vi "Insert_Into_Array_2D.vi"(9 "SubArray IIA 2D":i8[][](array[numeric]), 10 "Indexs IIA":T1, 11 "Insert Into Array 2D":i8[][](array[numeric])) -> (3 "Array 2D IIA":i8[][](array[numeric]))   [LabVIEW 2018]
uses:
  Controls/Rows_Columns.ctl
panel:
  out "IRR":i32
  out "ICC":i32
  out "SC":i32
  out "SR":i32
  out "IRC":i32
  out "SC1":i32
  out "SR1":i32
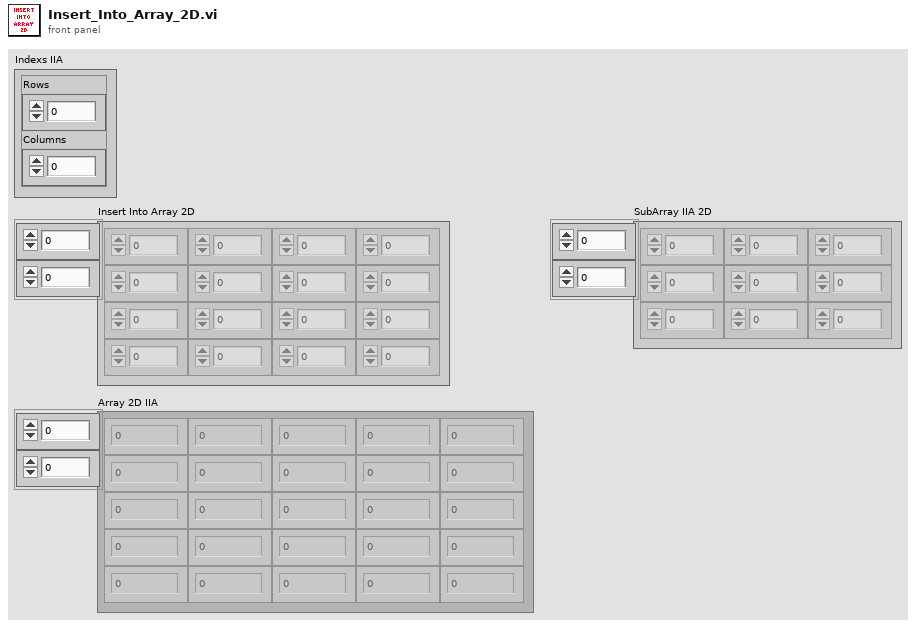
[diagram p1: front panel]
types:
  T1 = typedef "Rows_Columns.ctl" = cluster{"Rows":i32, "Columns":i32}
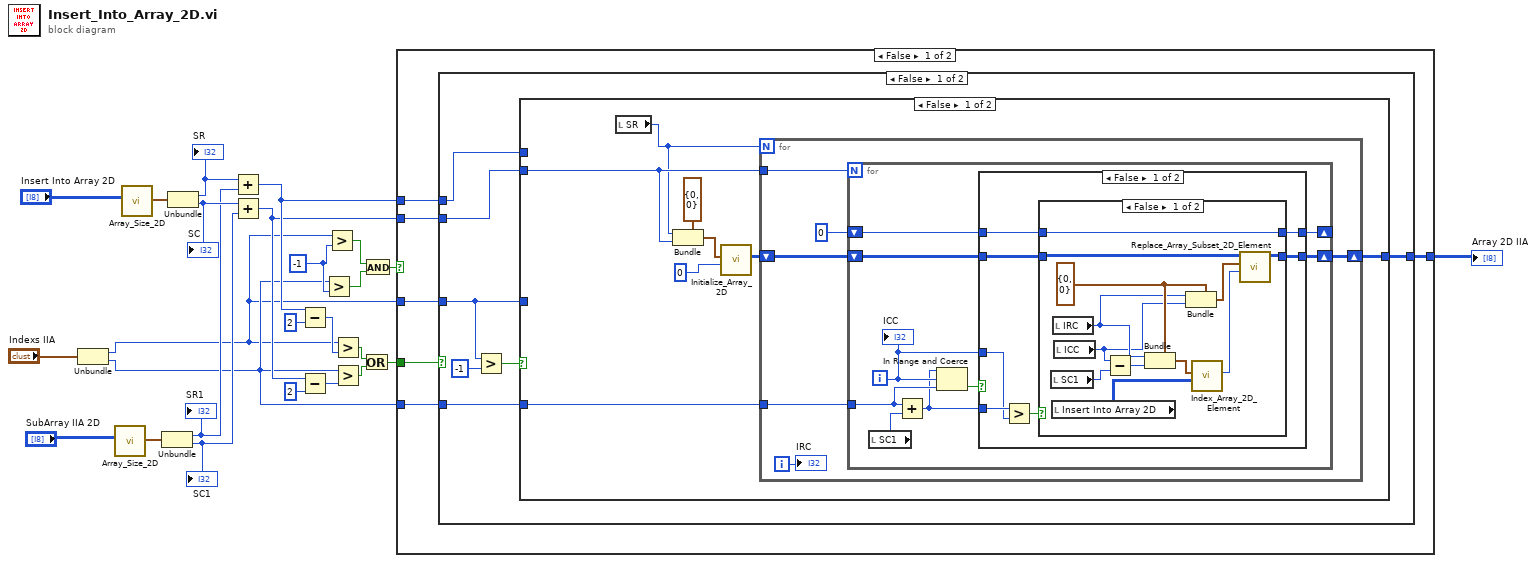
[diagram p0: block diagram]
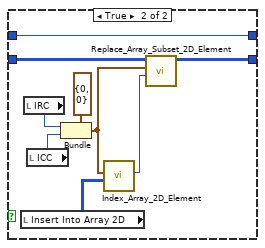
[diagram p2: hidden frame]
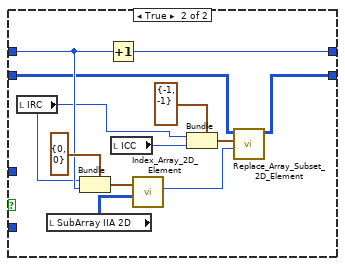
[diagram p3: hidden frame]
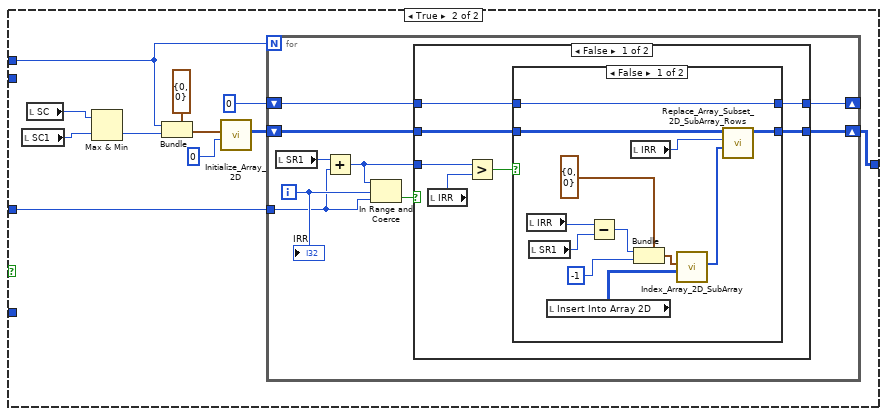
[diagram p4: hidden frame]
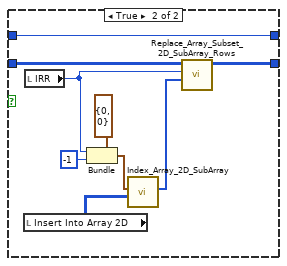
[diagram p5: hidden frame]
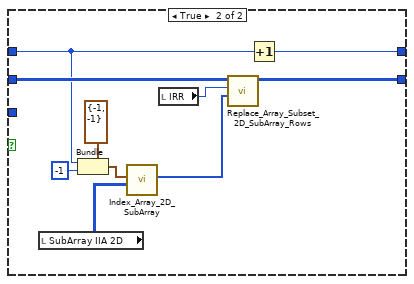
[diagram p6: hidden frame]
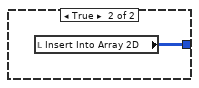
[diagram p7: hidden frame]
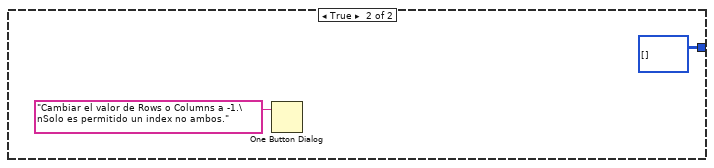
[diagram p8: hidden frame]
diagram:
  w3 = -1 ("y")
  n1 = Unbundle("Indexs IIA") -> ("Rows"=w1:i32, "Columns"=w2:i32)
  n2 = call "Array_Size_2D.vi"("Array"="SubArray IIA 2D") -> ("Size 2D"=w23:T1)  [unwired: 10 in]
  n3 = call "Array_Size_2D.vi"("Array"="Insert Into Array 2D") -> ("Size 2D"=w24:T1)  [unwired: 10 in]
  n4 = Unbundle(w23) -> ("Rows"=w10:i32, "Columns"=w21:i32)
  "SR1" <- w10
  "SC1" <- w21
  n5 = Unbundle(w24) -> ("Rows"=w11:i32, "Columns"=w22:i32)
  "SR" <- w11
  "SC" <- w22
  n6 = Add(x=w11, y=w10) -> (x+y=w18:i32)
  n7 = Add(x=w22, y=w21) -> (x+y=w9:i32)
  n8 = Subtract(x=w18, y=2) -> (x-y=w16:i32)
  n9 = Subtract(x=w9, y=2) -> (x-y=w14:i32)
  n10 = Greater?(x=w2, y=w3) -> (0:w4:bool)
  n11 = Greater?(x=w1, y=w3) -> (0:w5:bool)
  n12 = Greater?(x=w1, y=w16) -> (0:w20:bool)
  n13 = Greater?(x=w2, y=w14) -> (0:w19:bool)
  n14 = Or(x=w20, y=w19) -> (x .or. y?=w12:bool)
  n15 = And(x=w5, y=w4) -> (x .and. y?=w6:bool)
  n16 = case shown="False" w6 {
    tunnel: w18 -> [w31 _]
    tunnel: w12 -> [w30 _]
    tunnel: w9 -> [w29 _]
    tunnel: w2 -> [w28 _]
    tunnel: w1 -> [w27 _]
    tunnel: [w26 i8[][] [] ("Insert Into Array 2D")] -> w7
    frame False {
      n17 = case shown="False" w30 {
        tunnel: w31 -> [w35 _]
        tunnel: w27 -> [w33 _]
        tunnel: w28 -> [w34 _]
        tunnel: w29 -> [w36 _]
        tunnel: [w32 w160] -> w26
        frame False {
          n18 = Greater?(x=w33, y=-1) -> (0:w37:bool)
          n19 = case shown="False" w37 {
            tunnel: w36 -> [w45 _]
            tunnel: w35 -> [_ w106]
            tunnel: w34 -> [w46 _]
            tunnel: w33 -> [_ w108]
            tunnel: [w40 w105] -> w32
            frame False {
              n20 = local read "SR"() -> (w39:i32)
              n21 = Bundle(cluster=T1 {"Rows"=0, "Columns"=0} ("Dimensions"), "Rows"=w39, "Columns"=w45) -> (w42:T1)
              n22 = call "Initialize_Array_2D.vi"("Value"=i8 0, "Dimensions"=w42) -> ("Initialized Array 2D"=w41:i8[][])  [unwired: 9 in]
              n23 = for {
                N: w39 -> [_]
                tunnel: w45 -> [w51]
                shift-right: [w47] -> w40
                shift-left: w41 -> [w49]
                tunnel: w46 -> [w50]
                i -> [w52]
                n24 = for {
                  N: w51 -> [_]
                  tunnel: w50 -> [w61]
                  shift-right: [w55] -> _
                  shift-left: 0 -> [w56]
                  shift-right: [w53] -> w47
                  shift-left: w49 -> [w54]
                  i -> [w58]
                  n25 = local read "SC1"() -> (w60:i32)
                  n26 = Add(x=w61, y=w60) -> (x+y=w57:i32)
                  n27 = In Range and Coerce(upper limit=w57, x=w58, lower limit=w61) -> (In Range?=w59:bool)  [unwired: 1 out]
                  n28 = case shown="False" w59 {
                    tunnel: w58 -> [w67 _]
                    tunnel: w57 -> [w68 _]
                    tunnel: [w64 w101] -> w55
                    tunnel: w56 -> [w65 w99]
                    tunnel: w54 -> [w62 w94]
                    tunnel: [w63 w95] -> w53
                    frame False {
                      n29 = Greater?(x=w68, y=w67) -> (0:w66:bool)
                      n30 = case shown="False" w66 {
                        tunnel: [w80 w89] -> w64
                        tunnel: w65 -> [w80 w89]
                        tunnel: [w79 w88] -> w63
                        tunnel: w62 -> [w78 w87]
                        frame False {
                          w74 = T1 {"Rows"=0, "Columns"=0} ("Indexs IA")
                          n31 = local read "SC1"() -> (w72:i32)
                          n32 = local read "Insert Into Array 2D"() -> (w77:i8[][])
                          n33 = local read "IRC"() -> (w73:i32)
                          n34 = local read "ICC"() -> (w70:i32)
                          n35 = Subtract(x=w70, y=w72) -> (x-y=w71:i32)
                          n36 = Bundle(cluster=w74, "Rows"=w73, "Columns"=w71) -> (w69:T1)
                          n37 = Bundle(cluster=w74, "Rows"=w73, "Columns"=w70) -> (w75:T1)
                          n38 = call "Index_Array_2D_Element.vi"("Index Array 2D"=w77, "Indexs IA"=w69) -> ("Value"=w76:i8)  [unwired: 9 in]
                          n39 = call "Replace_Array_Subset_2D_Element.vi"("Element RAS"=w76, "Indexs RAS"=w75, "RAS2D"=w78) -> ("New Array RAS2D"=w79:i8[][])  [unwired: 8 in]
                        }
                        frame True {
                          n40 = local read "Insert Into Array 2D"() -> (w85:i8[][])
                          n41 = local read "IRC"() -> (w82:i32)
                          n42 = local read "ICC"() -> (w83:i32)
                          n43 = Bundle(cluster=T1 {"Rows"=0, "Columns"=0} ("Indexs IA"), "Rows"=w82, "Columns"=w83) -> (w81:T1)
                          n44 = call "Index_Array_2D_Element.vi"("Index Array 2D"=w85, "Indexs IA"=w81) -> ("Value"=w86:i8)  [unwired: 9 in]
                          n45 = call "Replace_Array_Subset_2D_Element.vi"("Element RAS"=w86, "Indexs RAS"=w81, "RAS2D"=w87) -> ("New Array RAS2D"=w88:i8[][])  [unwired: 8 in]
                        }
                      }
                    }
                    frame True {
                      n46 = local read "IRC"() -> (w90:i32)
                      n47 = local read "SubArray IIA 2D"() -> (w97:i8[][])
                      n48 = Bundle(cluster=T1 {"Rows"=0, "Columns"=0} ("Indexs IA"), "Rows"=w90, "Columns"=w99) -> (w98:T1)
                      n49 = Increment(x=w99) -> (x+1=w101:i32)
                      n50 = local read "ICC"() -> (w91:i32)
                      n51 = call "Index_Array_2D_Element.vi"("Index Array 2D"=w97, "Indexs IA"=w98) -> ("Value"=w96:i8)  [unwired: 9 in]
                      n52 = Bundle(cluster=T1 {"Rows"=-1, "Columns"=-1} ("Rows & Columns"), "Rows"=w90, "Columns"=w91) -> (w92:T1)
                      n53 = call "Replace_Array_Subset_2D_Element.vi"("Element RAS"=w96, "Indexs RAS"=w92, "RAS2D"=w94) -> ("New Array RAS2D"=w95:i8[][])  [unwired: 8 in]
                    }
                  }
                  "ICC" <- w58
                }
                "IRC" <- w52
              }
            }
            frame True {
              n54 = local read "SC1"() -> (w103:i32)
              n55 = local read "SC"() -> (w104:i32)
              n56 = Max & Min(x=w104, y=w103) -> (min(x,y)=w102:i32)  [unwired: 1 out]
              n57 = Bundle(cluster=T1 {"Rows"=0, "Columns"=0} ("Dimensions"), "Rows"=w106, "Columns"=w102) -> (w111:T1)
              n58 = call "Initialize_Array_2D.vi"("Value"=i8 0, "Dimensions"=w111) -> ("Initialized Array 2D"=w109:i8[][])  [unwired: 9 in]
              n59 = for {
                N: w106 -> [_]
                tunnel: w108 -> [w120]
                shift-right: [w114] -> _
                shift-left: 0 ("Value") -> [w118]
                shift-right: [w115] -> w105
                shift-left: w109 -> [w116]
                i -> [w121]
                n60 = local read "SR1"() -> (w119:i32)
                n61 = Add(x=w119, y=w120) -> (x+y=w113:i32)
                n62 = In Range and Coerce(upper limit=w113, x=w121, lower limit=w120) -> (In Range?=w117:bool)  [unwired: 1 out]
                n63 = case shown="False" w117 {
                  tunnel: w118 -> [w122 w151]
                  tunnel: w116 -> [w125 w155]
                  tunnel: [w124 w152] -> w115
                  tunnel: [w123 w150] -> w114
                  tunnel: w113 -> [w127 _]
                  frame False {
                    n64 = local read "IRR"() -> (w128:i32)
                    n65 = Greater?(x=w127, y=w128) -> (0:w126:bool)
                    n66 = case shown="False" w126 {
                      tunnel: w125 -> [w136 w148]
                      tunnel: [w135 w147] -> w124
                      tunnel: [w140 w146] -> w123
                      tunnel: w122 -> [w140 w146]
                      frame False {
                        n67 = local read "IRR"() -> (w131:i32)
                        n68 = local read "SR1"() -> (w130:i32)
                        n69 = local read "Insert Into Array 2D"() -> (w139:i8[][])
                        n70 = Subtract(x=w131, y=w130) -> (x-y=w132:i32)
                        n71 = local read "IRR"() -> (w129:i32)
                        n72 = Bundle(cluster=T1 {"Rows"=0, "Columns"=0} ("Indexs IA"), "Rows"=w132, "Columns"=-1) -> (w133:T1)
                        n73 = call "Index_Array_2D_SubArray.vi"("Index Array 2D"=w139, "Indexs IA"=w133) -> ("Index SubArray"=w134:i8[])  [unwired: 9 in]
                        n74 = call "Replace_Array_Subset_2D_SubArray_Rows.vi"("SubArray RAS2D"=w134, "Index Row"=w129, "RAS2D"=w136) -> ("New Array RAS2D"=w135:i8[][])  [unwired: 8 in]
                      }
                      frame True {
                        n75 = local read "Insert Into Array 2D"() -> (w145:i8[][])
                        n76 = local read "IRR"() -> (w141:i32)
                        n77 = Bundle(cluster=T1 {"Rows"=0, "Columns"=0} ("Indexs IA"), "Rows"=w141, "Columns"=-1) -> (w143:T1)
                        n78 = call "Index_Array_2D_SubArray.vi"("Index Array 2D"=w145, "Indexs IA"=w143) -> ("Index SubArray"=w149:i8[])  [unwired: 9 in]
                        n79 = call "Replace_Array_Subset_2D_SubArray_Rows.vi"("SubArray RAS2D"=w149, "Index Row"=w141, "RAS2D"=w148) -> ("New Array RAS2D"=w147:i8[][])  [unwired: 8 in]
                      }
                    }
                  }
                  frame True {
                    n80 = local read "SubArray IIA 2D"() -> (w159:i8[][])
                    n81 = Bundle(cluster=T1 {"Rows"=-1, "Columns"=-1} ("Indexs IA"), "Rows"=w151, "Columns"=-1) -> (w157:T1)
                    n82 = call "Index_Array_2D_SubArray.vi"("Index Array 2D"=w159, "Indexs IA"=w157) -> ("Index SubArray"=w153:i8[])  [unwired: 9 in]
                    n83 = local read "IRR"() -> (w154:i32)
                    n84 = call "Replace_Array_Subset_2D_SubArray_Rows.vi"("SubArray RAS2D"=w153, "Index Row"=w154, "RAS2D"=w155) -> ("New Array RAS2D"=w152:i8[][])  [unwired: 8 in]
                    n85 = Increment(x=w151) -> (x+1=w150:i32)
                  }
                }
                "IRR" <- w121
              }
            }
          }
        }
        frame True {
          n86 = local read "Insert Into Array 2D"() -> (w160:i8[][])
        }
      }
    }
    frame True {
      n87 = One Button Dialog(message="Cambiar el valor de Rows o Columns a -1.\nSolo es permitido un index no ambos.") -> ()  [unwired: 1 in, 1 out]
    }
  }
  "Array 2D IIA" <- w7
